vi "read_settings_file.vi"(8 "error in (no error)":errorcluster, 9 "settings cluster in":variant, 10 "settings name":string, 11 "ScanModeTS090821Circular2D in":refnum<class "ImagingModeTS090821Circular2D.lvclass">) -> (0 "error out":errorcluster, 1 "settings cluster out":variant, 3 "ScanModeTS090821Circular2D out":refnum<class "ImagingModeTS090821Circular2D.lvclass">)   [LabVIEW 2010, in "ImagingModeTS090821Circular2D.lvclass"]
uses:
  ImagingModeTS090821Circular2D.lvclass
  ImagingModeDL091001Scaffold/ImagingModeDL091001Scaffold/ImagingModeDL091001Scaffold.lvclass
  ImagingModeTS090821Circular2D.lvclass/ImagingModeTS090821Circular2D.ctl
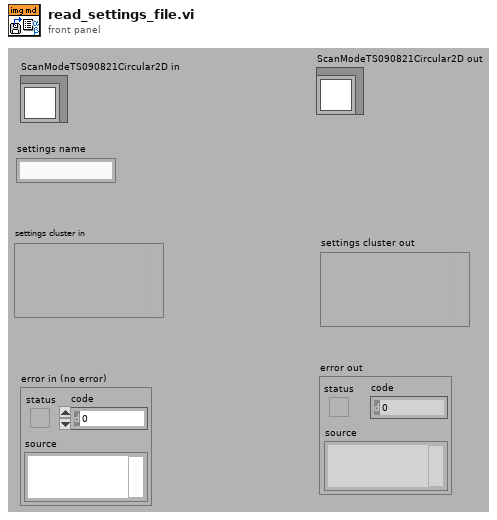
[diagram p1: front panel]
types:
  T1 = typedef "ImagingModeTS090821Circular2D.lvclass/settings_cluster.ctl" = cluster{"AmplitudeX":dbl[unit], "AmplitudeY":dbl[unit], "FrequencyY":dbl, "FrequencyX":dbl, "PhaseShift":dbl, "CenterX":dbl, "CenterY":dbl, "RotationAngle":dbl, "ScanRate":dbl[unit], "Spiral":bool, "DumpFactor":dbl, "TotalPixelsPerCycle":i32, "NumberOfCycles":i32, "LinesPerFrame":i32, "Double":bool}
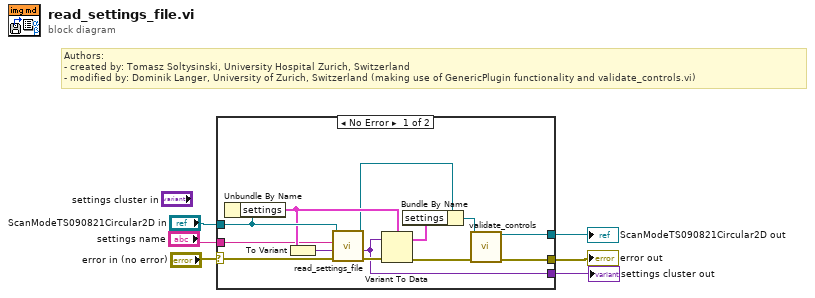
[diagram p0: block diagram]
diagram:
  # "Authors: \n- created by: Tomasz Soltysinski, University Hospital Zurich, Switzerland\n- modified by: Dominik Langer, University of Zurich, Switzerland (making use of GenericPlugin functionality and validate_controls.vi)"
  n1 = case shown="No Error" "error in (no error)" {
    selector: "error in (no error)" -> [w18 w21]
    tunnel: [w8 w21] -> w3
    tunnel: [w9 w20] -> w5
    tunnel: "ScanModeTS090821Circular2D in" -> [w17 w20]
    tunnel: "settings name" -> [w14 _]
    tunnel: [w7 _] -> w1
    frame No Error {
      n2 = Unbundle By Name(w17) -> ("settings"=w15:T1)
      n3 = To Variant(anything=w15) -> (Variant=w16:variant)
      n4 = call-parent "read_settings_file.vi"("error in (no error)"=w18, "settings cluster in"=w16, "settings name"=w14, "GenericPlugin in"=w17) -> ("error out"=w19:errorcluster, "settings cluster out"=w7:variant, "GenericPlugin out"=w10:refnum<class "ImagingModeTS090821Circular2D.lvclass">)  [unwired: 5 in]
      n5 = Variant To Data(error in=w19, Variant=w7, type=w15) -> (error out=w13:errorcluster, data=w12:T1)
      n6 = Bundle By Name(cluster=w10, "settings"=w12) -> (w11:refnum<class "ImagingModeTS090821Circular2D.lvclass">)
      n7 = call-dynamic "validate_controls.vi"("error in (no error)"=w13, "ScanModeTS090821Circular2D in"=w11) -> ("error out"=w8:errorcluster, "ScanModeTS090821Circular2D out"=w9:refnum<class "ImagingModeTS090821Circular2D.lvclass">)  [unwired: 8 in]
    }
    frame Error {
    }
  }
  "ScanModeTS090821Circular2D out" <- w5
  "error out" <- w3
  "settings cluster out" <- w1
